vi "get all US data.vi"() -> (1 "populations":i32[](array[numeric]), 2 "cases countries":string[](array[string]), 3 "US data":T1)   [LabVIEW 2019]
panel:
  out "x = y?":bool
  out "deaths countries":string[](array[string])
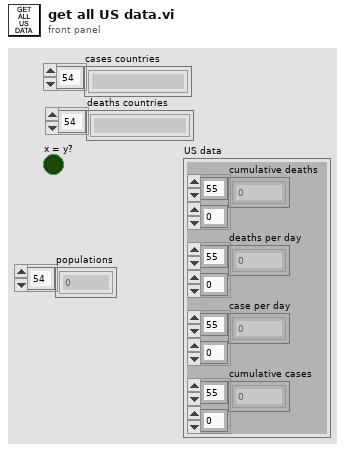
[diagram p1: front panel]
types:
  T1 = cluster{"cumulative deaths":i32[][], "deaths per day":i32[][], "case per day":i32[][], "cumulative cases":i32[][]}
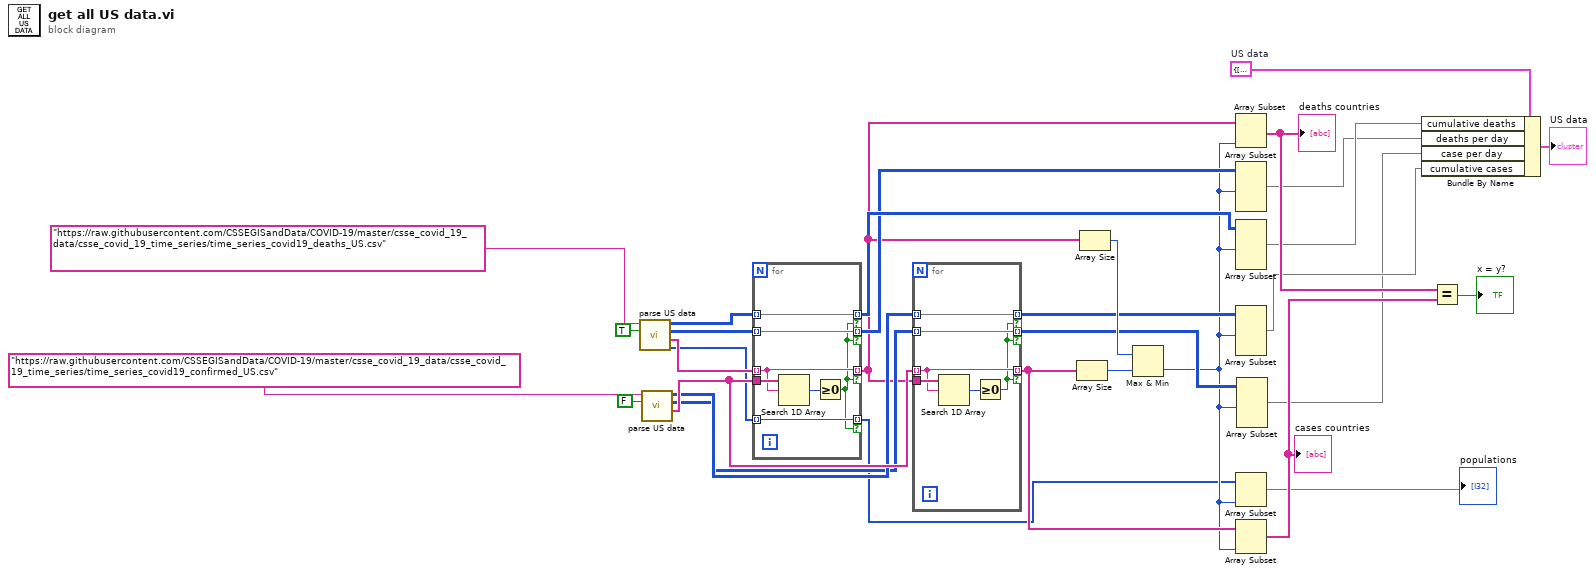
[diagram p0: block diagram]
diagram:
  w9 = T1 {"cumulative deaths"=[], "deaths per day"=[], "case per day"=[], "cumulative cases"=[]}  # US data
  n1 = call "parse US data.vi"("has population values"=TRUE, "String"="https://raw.githubusercontent.com/CSSEGISandData/COVID-19/master/csse_covid_19_data/csse_covid_19_time_series/time_series_covid19_deaths_US.csv") -> ("populations"=w2:i32[], "Array 3"=w27:string[], "per day"=w25:i32[][], "cumulative"=w26:i32[][])  [unwired: 6 in]
  n2 = call "parse US data.vi"("has population values"=FALSE, "String"="https://raw.githubusercontent.com/CSSEGISandData/COVID-19/master/csse_covid_19_data/csse_covid_19_time_series/time_series_covid19_confirmed_US.csv") -> ("Array 3"=w24:string[], "per day"=w22:i32[][], "cumulative"=w23:i32[][])  [unwired: 6 in, 1 out]
  n3 = for {
    tunnel: w27 -> [w34] mode=indexing
    tunnel: w24 -> [w38]
    tunnel: w26 -> [w37] mode=indexing
    tunnel: w25 -> [w36] mode=indexing
    tunnel: [w37] -> w16 mode=indexing if=w32
    tunnel: [w36] -> w15 mode=indexing if=w32
    tunnel: [w34] -> w14 mode=indexing if=w32
    tunnel: w2 -> [w33] mode=indexing
    tunnel: [w33] -> w1 mode=indexing if=w32
    n4 = Search 1D Array(1D array=w38, element=w34) -> (index of element=w35:i32)  [unwired: 1 in]
    n5 = Greater Or Equal To 0?(x=w35) -> (x >= 0?=w32:bool)
  }
  n6 = for {
    tunnel: w24 -> [w40] mode=indexing
    tunnel: w14 -> [w44]
    tunnel: w23 -> [w43] mode=indexing
    tunnel: w22 -> [w42] mode=indexing
    tunnel: [w43] -> w17 mode=indexing if=w39
    tunnel: [w42] -> w18 mode=indexing if=w39
    tunnel: [w40] -> w13 mode=indexing if=w39
    n7 = Search 1D Array(1D array=w44, element=w40) -> (index of element=w41:i32)  [unwired: 1 in]
    n8 = Greater Or Equal To 0?(x=w41) -> (x >= 0?=w39:bool)
  }
  n9 = Array Size(array=w13) -> (size(s)=w20:i32)
  n10 = Array Size(array=w14) -> (size(s)=w19:i32)
  n11 = Max & Min(x=w19, y=w20) -> (min(x,y)=w12:i32)  [unwired: 1 out]
  n12 = Array Subset(array=w14, length=w12) -> (w10:string[])  [unwired: 1 in]
  "deaths countries" <- w10
  n13 = Array Subset(array=w15, length (row)=w12) -> (w7:i32[][])  [unwired: 3 in]
  n14 = Array Subset(array=w16, length (row)=w12) -> (w8:i32[][])  [unwired: 3 in]
  n15 = Array Subset(array=w17, length (row)=w12) -> (w6:i32[][])  [unwired: 3 in]
  n16 = Array Subset(array=w1, length=w12) -> (→"populations":i32[])  [unwired: 1 in]
  n17 = Array Subset(array=w13, length=w12) -> (w11:string[])  [unwired: 1 in]
  "cases countries" <- w11
  n18 = Array Subset(array=w18, length (row)=w12) -> (w5:i32[][])  [unwired: 3 in]
  n19 = Bundle By Name(cluster=w9, "cumulative deaths"=w8, "deaths per day"=w7, "case per day"=w5, "cumulative cases"=w6) -> (→"US data":T1)
  n20 = Equal?(x=w10, y=w11) -> (x = y?=→"x = y?":bool)
